vi "차량좌표계.vi"(2 "GPS":dbl[][](array[numeric])) -> (5 "Upper Boundary":dbl[][](array[numeric]), 6 "Lower Boundary":dbl[][](array[numeric]), 7 "Left Boundary":dbl[][](array[numeric]), 8 "Right Boundary":dbl[][](array[numeric]))   [LabVIEW 2016]
uses:
  <vilib>/imath/engines/lvmath2/RunTimeEngine/Managers/WorkSpace/UID Generator.vi
  <vilib>/imath/engines/lvmath2/RunTimeEngine/RunTimeType/NIMS_RunTimeType_From StrictType (excl LVString).vi
  <instcachedir>/0/NIMS_RunTimeType_From StrictType (excl LVString)_BBF44FB49F834B71AF7A14CCEDF8BECD.lvgen/NIMS_RunTimeType_From StrictType (excl LVString)_BBF44FB49F834B71AF7A14CCEDF8BECD_000.vi
  <vilib>/imath/engines/lvmath2/RunTimeEngine/LocalVariableDefStatement/MC_LocalVariableDefStatement_Display.vi
  <vilib>/imath/engines/lvmath2/RunTimeEngine/IndexRead/NIMS M(S).vi
  <instcachedir>/0/NIMS M(S)_B826C018497E4940AE96BD27B540B6FB.lvgen/NIMS M(S)_B826C018497E4940AE96BD27B540B6FB_000.vi
  <vilib>/imathl/engines/lvmath/Functions/Error Handling/Create Error.vi
  <vilib>/imath/engines/lvmath2/RunTimeEngine/BuiltInFunctions/deg_to_rad/NIMS_deg_to_rad.vi
  <instcachedir>/0/NIMS_deg_to_rad_4A81D684CE8D4DD79924F5AB74D756E1.lvgen/NIMS_deg_to_rad_4A81D684CE8D4DD79924F5AB74D756E1_001.vi
  <vilib>/imath/engines/lvmath2/RunTimeEngine/RangeToken/NIMS_Range.vi
  <instcachedir>/0/NIMS_Range_A7C094595B484CA7AF10685B02D808ED.lvgen/NIMS_Range_A7C094595B484CA7AF10685B02D808ED_000.vi
  <vilib>/imath/engines/lvmath2/RunTimeEngine/ArithmeticOperatorToken/NIMS_ArithmeticOperator_rightdiv.vi
  <instcachedir>/0/NIMS_ArithmeticOperator_rightdiv_0403F5D95ED04A4080FE3DA43A6A83B7.lvgen/NIMS_ArithmeticOperator_rightdiv_0403F5D95ED04A4080FE3DA43A6A83B7_000.vi
  <vilib>/imath/engines/lvmath2/RunTimeEngine/RowToken/NIMS_RowToken_CV_CV.vi
  <instcachedir>/0/NIMS_RowToken_CV_CV_5546A0B1CA2C4E49826F811B9C073FB0.lvgen/NIMS_RowToken_CV_CV_5546A0B1CA2C4E49826F811B9C073FB0_000.vi
  <vilib>/imath/engines/lvmath2/RunTimeEngine/ArithmeticOperatorToken/NIMS_ArithmeticOperator_multmx-internal.vi
  <instcachedir>/0/NIMS_ArithmeticOperator_multmx-internal_EB2A2C7A937F4195916A6EDDDE2C7733.lvgen/NIMS_ArithmeticOperator_multmx-internal_EB2A2C7A937F4195916A6EDDDE2C7733_004.vi
  <vilib>/imath/engines/lvmath2/RunTimeEngine/ErrorHandling/NIMS_Create Error From Enums.vi
  <vilib>/imath/engines/lvmath2/RunTimeEngine/ArithmeticOperatorToken/NIMS_ArithmeticOperator_plus.vi
  <instcachedir>/0/NIMS_ArithmeticOperator_plus_0120E0498A0F4B4B9BDCAC2554767A4E.lvgen/NIMS_ArithmeticOperator_plus_0120E0498A0F4B4B9BDCAC2554767A4E_003.vi
  <vilib>/imath/engines/lvmath2/RunTimeEngine/Managers/SymbolTable/Clear UID.vi
  <vilib>/imath/engines/lvmath2/RunTimeEngine/NodeEndStatement/NIMS_NodeEndStatement_Output.vi
  <instcachedir>/0/NIMS_NodeEndStatement_Output_53EC0D466D134D7ABD903AC30B43404B.lvgen/NIMS_NodeEndStatement_Output_53EC0D466D134D7ABD903AC30B43404B_002.vi
  <vilib>/imath/engines/lvmath2/RunTimeEngine/ErrorHandling/NIMS_Finalize Error.vi
  <vilib>/imath/engines/lvmath2/RunTimeEngine/Managers/SymbolTable/NIMS_WorkSpace.lvlib
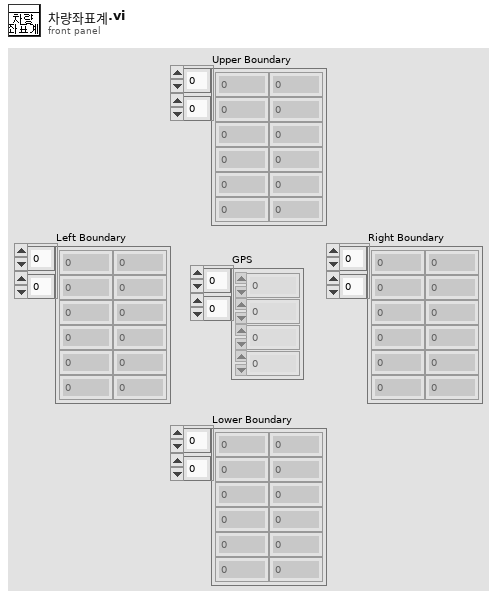
[diagram p1: front panel]
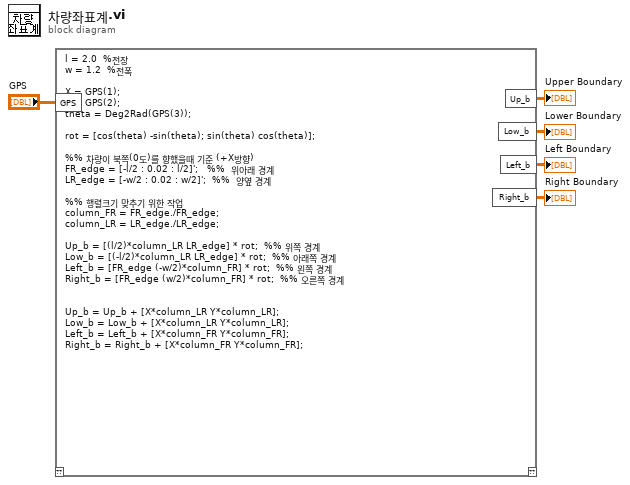
[diagram p0: block diagram]
diagram:
  n1 = mathscript code="l = 2.0  %전장\nw = 1.2  %전폭\n\nX = GPS(1);\nY = GPS(2);\ntheta = Deg2Rad(GPS(3));\n\nrot = [cos(theta) -sin(theta); sin(theta) cos(theta)];\n\n%% 차량이 북쪽(0도)를 향했을때 기준 (+X방향)\nFR_edge = [-l/2 : 0.02 : l/2]';   %%  위아래 경계\nLR_edge = [-w/2 : 0.02 : w/2]';  %%  양옆 경계\n\n%% 행렬크기 맞추기 위한 작업\ncolumn_FR = FR_edge./FR_edge;\ncolumn_LR = LR_edge./LR_edge;\n\nUp_b = [(l/2)*column_LR LR_edge] * rot;  %% 위쪽 경계\nLow_b = [(-l/2)*column_LR LR_edge] * rot;  %% 아래쪽 경계\nLeft_b = [FR_edge (-w/2)*column_FR] * rot;  %% 왼쪽 경계\nRight_b = [FR_edge (w/2)*column_FR] * rot;  %% 오른쪽 경계\n\n\nUp_b = Up_b + [X*column_LR Y*column_LR];\nLow_b = Low_b + [X*column_LR Y*column_LR];\nLeft_b = Left_b + [X*column_FR Y*column_FR];\nRight_b = Right_b + [X*column_FR Y*column_FR];"("GPS"="GPS") -> ("Up_b"=→"Upper Boundary":dbl[][], "Low_b"=→"Lower Boundary":dbl[][], "Left_b"=→"Left Boundary":dbl[][], "Right_b"=→"Right Boundary":dbl[][])  [unwired: 1 in, 1 out]
